vi "PicoScope2000aGetStreamingValues.vi"(10 "handle in":i16, 11 "error in":errorcluster) -> (0 "Start Index":u32, 1 "Trigger":cluster{bool, "triggeredAt":u32}, 2 "handle out":i16, 3 "error out":errorcluster, 4 "Number of Samples":i32, 5 "ready":i16, 6 "Auto Stopped":bool)   [LabVIEW 2010]
doc: "This VI is used in streaming mode to get the latest values from the driver. It should be called in a loop after the oscilloscope has been set up using PicoScope3000aSettings.vi and streaming has been started by calling PicoScope3000aStartStreaming.vi. The VI outputs the number of samples available and the start index of these samples in the array output by PicoScope3000aStartStreaming.vi."
uses:
  ps2000aWrap.dll
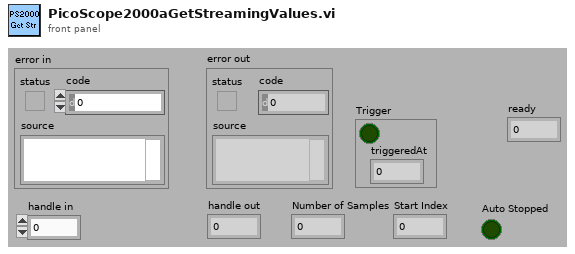
[diagram p1: front panel]
types:
  T1 = cluster{"status":bool, "code":u32, "source":string}
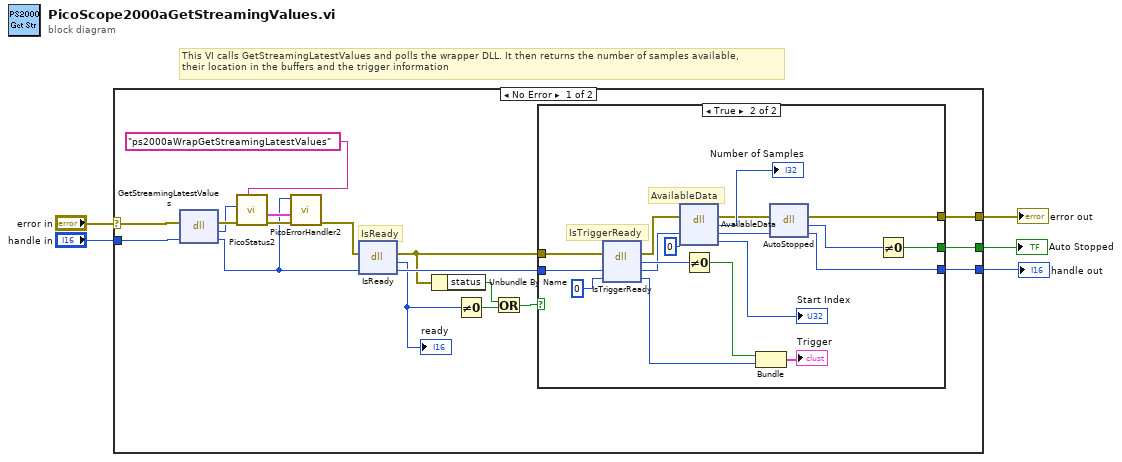
[diagram p0: block diagram]
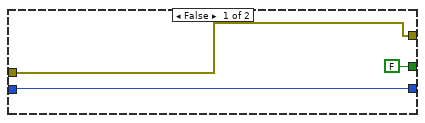
[diagram p2: hidden frame]
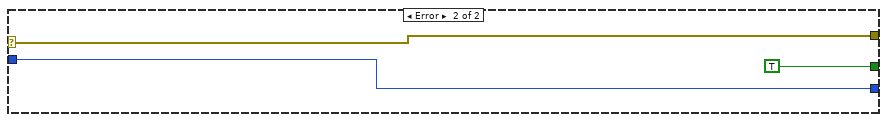
[diagram p3: hidden frame]
diagram:
  # "This VI calls GetStreamingLatestValues and polls the wrapper DLL. It then returns the number of samples available, \ntheir location in the buffers and the trigger information"
  n1 = case shown="No Error" "error in" {
    selector: "error in" -> [w22 w47]
    tunnel: [w6 w47] -> w4
    tunnel: "handle in" -> [w23 w46]
    tunnel: [w10 w46] -> w2
    tunnel: [w19 TRUE] -> w1
    frame No Error {
      # "IsReady"
      n2 = dll-call lib="ps2000aWrap.dll" fn="GetStreamingLatestValues" ("PS5000.dll:_ps5000SetDataBuffer@16")(error in=w22, "handle"=w23) -> (error out=w17:errorcluster, "PICO_STATUS"=w16:u32, "handle"=w8:i16)  [unwired: 2 in, 1 out]
      n3 = call "PicoStatus2.vi"("PICO source"="ps2000aWrapGetStreamingLatestValues" ("source"), "Error in"=w17, "PICO STATUS"=w16) -> ("error out"=w9:errorcluster, "PICO_STATUS out"=w11:T1)  [unwired: 5 in]
      n4 = call "PicoErrorHandler2.vi"("error in (no error)"=w9, "PICO_STATUS in"=w11, "handle In"=w8) -> ("error out"=w7:errorcluster)  [unwired: 8 in]
      n5 = dll-call lib="ps2000aWrap.dll" fn="IsReady" ("PS5000.dll:_ps5000SetDataBuffer@16")(error in=w7, "handle"=w8) -> (error out=w20:errorcluster, "ready"=w13:i16, "handle"=w21:i16)  [unwired: 2 in, 1 out]
      "ready" <- w13
      n6 = Unbundle By Name(w20) -> ("status"=w14:bool)
      n7 = Not Equal To 0?(x=w13) -> (x != 0?=w18:bool)
      n8 = Or(x=w14, y=w18) -> (x .or. y?=w12:bool)
      n9 = case shown="True" w12 {
        tunnel: [w26 w27] -> w6
        tunnel: w21 -> [w25 w43]
        tunnel: w20 -> [w26 w37]
        tunnel: [FALSE w32] -> w19
        tunnel: [w25 w28] -> w10
        frame False {
        }
        frame True {
          # "AvailableData"
          # "IsTriggerReady"
          n10 = dll-call lib="ps2000aWrap.dll" fn="IsTriggerReady" ("PS5000.dll:_ps5000SetDataBuffer@16")(error in=w37, "handle"=w43, "triggeredAt"=u32 0) -> (error out=w38:errorcluster, "triggered"=w42:i16, "handle"=w30:i16, "triggeredAt"=w40:u32)  [unwired: 2 in, 1 out]
          n11 = dll-call lib="ps2000aWrap.dll" fn="AvailableData" ("PS5000.dll:_ps5000Stop@4")(error in=w38, "handle"=w30, "startIndex"=u32 0) -> (error out=w33:errorcluster, "numSamples"=→"Number of Samples":i32, "handle"=w29:i16, "startIndex"=→"Start Index":u32)  [unwired: 2 in, 1 out]
          n12 = Not Equal To 0?(x=w42) -> (x != 0?=w41:bool)
          n13 = Bundle(w41, "triggeredAt"=w40) -> (→"Trigger":cluster{bool, "triggeredAt":u32})  [unwired: 1 in]
          n14 = dll-call lib="ps2000aWrap.dll" fn="AutoStopped"(error in=w33, "handle"=w29) -> (error out=w27:errorcluster, "autoStopped"=w31:i16, "handle"=w28:i16)  [unwired: 2 in, 1 out]
          n15 = Not Equal To 0?(x=w31) -> (x != 0?=w32:bool)
        }
      }
    }
    frame Error {
    }
  }
  "error out" <- w4
  "handle out" <- w2
  "Auto Stopped" <- w1
